vi "Configure Modulation(OSK).vi"(0 "VISA resource name":refnum<visa-resource-name>, 1 "Enable OSK Modulation (F: Disable)":bool, 3 "Oscillate Period (0.0001 s)":dbl=0.0001, 5 "Channel (1: Channel 1)":i32(ring)=1 items=["Channel 1"=1, "Channel 2"=2], 9 "OSK Source (0: Internal)":i32(ring) items=["Internal", "External"], 11 "error in (no error)":errorcluster, 13 "OSK Rate (100 Hz)":dbl=100.0) -> (4 "VISA resource name out":refnum<visa-resource-name>, 15 "error out":errorcluster)   [LabVIEW 2012, in "RIGOL DG4000 Series.lvlib"]
doc: "Configures OSK (Oscillation Keying) modulation.\n\nNote:\nOSK is only available when Sine is enabled."
uses:
  <instrlib>/RIGOL DG4000 Series/RIGOL DG4000 Series.lvlib
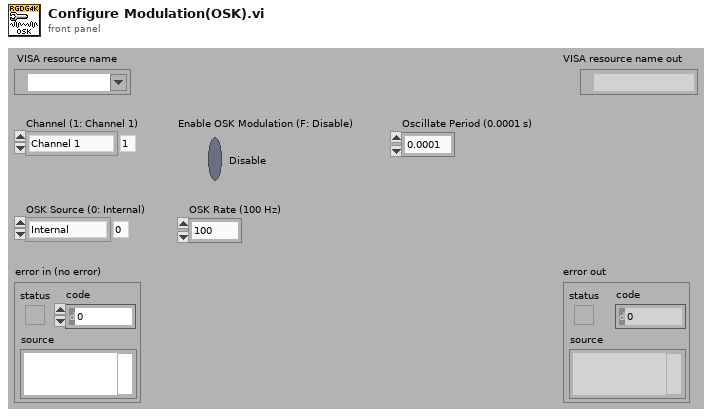
[diagram p1: front panel]
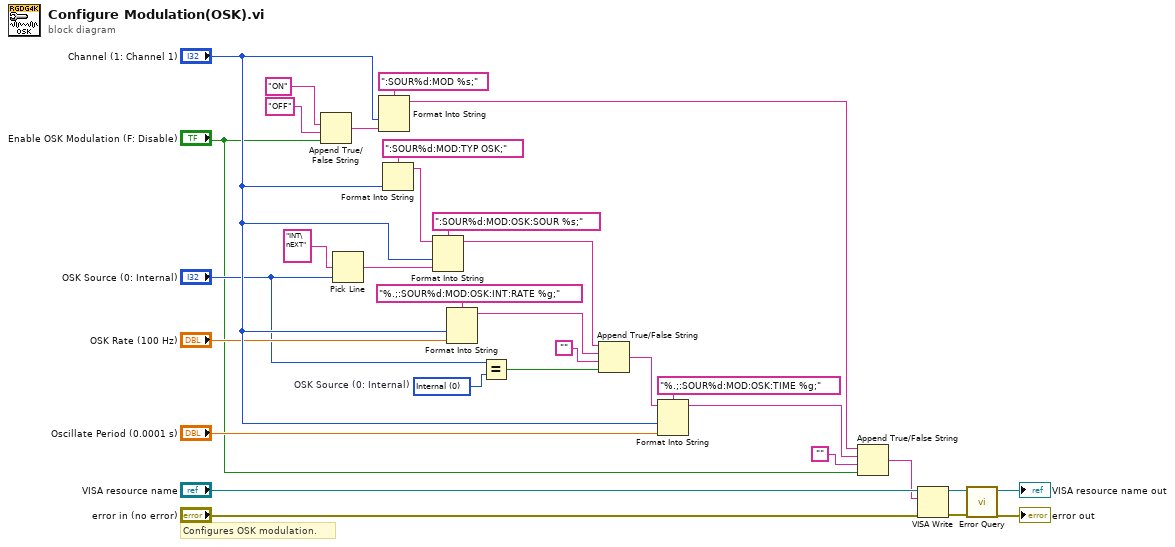
[diagram p0: block diagram]
diagram:
  w8 = 0 items=["Internal", "External"]  # OSK Source (0: Internal)
  # "Configures OSK modulation."
  n1 = Append True/False String(1:"Enable OSK Modulation (F: Disable)", 2:"OFF", 3:"ON") -> (0:w28:string)  [unwired: 1 out]
  n2 = Pick Line(multi-line string="INT\nEXT", line index="OSK Source (0: Internal)") -> (output string=w23:string)  [unwired: 1 out]
  n3 = Format Into String(format string=":SOUR%d:MOD %s;", "Channel (1: Channel 1)", w28) -> (resulting string=w2:string)  [unwired: 2 in, 1 out]
  n4 = Format Into String(format string=":SOUR%d:MOD:TYP OSK;", "Channel (1: Channel 1)") -> (resulting string=w25:string)  [unwired: 2 in, 1 out]
  n5 = Format Into String(format string=":SOUR%d:MOD:OSK:SOUR %s;", initial string=w25, "Channel (1: Channel 1)", w23) -> (resulting string=w12:string)  [unwired: 1 in, 1 out]
  n6 = Format Into String(format string="%.;:SOUR%d:MOD:OSK:INT:RATE %g;", "Channel (1: Channel 1)", "OSK Rate (100 Hz)") -> (resulting string=w10:string)  [unwired: 2 in, 1 out]
  n7 = Equal?(x="OSK Source (0: Internal)", y=w8) -> (x = y?=w9:bool)
  n8 = Append True/False String(1:w9, 2:"", 3:w10, 4:w12) -> (0:w6:string)
  n9 = Format Into String(format string="%.;:SOUR%d:MOD:OSK:TIME %g;", initial string=w6, "Channel (1: Channel 1)", "Oscillate Period (0.0001 s)") -> (resulting string=w1:string)  [unwired: 1 in, 1 out]
  n10 = Append True/False String(1:"Enable OSK Modulation (F: Disable)", 2:"", 3:w1, 4:w2) -> (0:w4:string)
  n11 = VISA Write(VISA resource name="VISA resource name", write buffer=w4, error in (no error)="error in (no error)") -> (VISA resource name out=w16:refnum<visa-resource-name>, error out=w15:errorcluster)  [unwired: 1 out]
  n12 = call <instrlib>:"Error Query.vi"("error in (no error)"=w15, "VISA resource name"=w16) -> ("error out"=→"error out":errorcluster, "VISA resource name out"=→"VISA resource name out":refnum<visa-resource-name>)  [unwired: 8 out]
